vi "MathCad_Matrix_Get_string Elmnt.vi"(4 "row":i32, 6 "col":i32, 7 "error in":errorcluster, 8 "Mathcad.IMatrixValue Refnum":refnum<k7>, 9 "Worksheet Reference In":refnum<k7>) -> (0 "error out":errorcluster, 2 "Mathcad.IMatrixValue Refnum":refnum<k7>, 3 "Worksheet Reference Out":refnum<k7>, 5 "string":string)   [LabVIEW 2015]
doc: "Gets the value from the reference retrieved from the getrefnum VI."
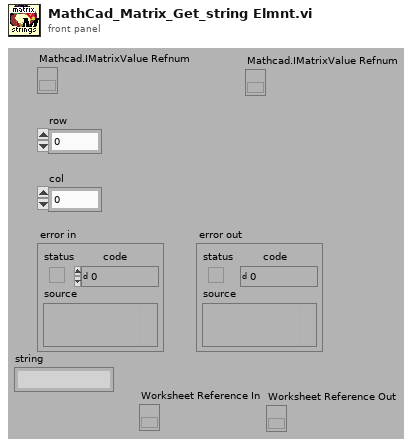
[diagram p1: front panel]
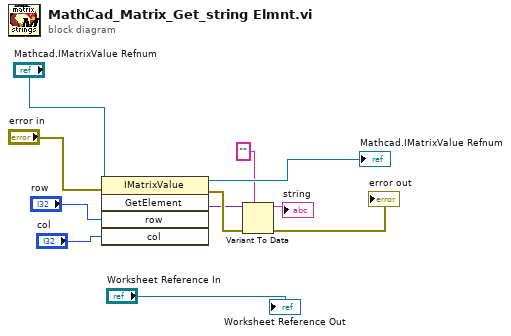
[diagram p0: block diagram]
diagram:
  n1 = invoke class="IMatrixValue" method="GetElement"(reference="Mathcad.IMatrixValue Refnum", error in="error in", "row"="row", "col"="col") -> (reference out=→"Mathcad.IMatrixValue Refnum":refnum<k7>, error out=w9:errorcluster, "GetElement"=w8:variant)  [unwired: 1 in, 2 out]
  n2 = Variant To Data(error in=w9, type="" ("data"), Variant=w8) -> (data=→"string":string, error out=→"error out":errorcluster)
  "Worksheet Reference Out" <- "Worksheet Reference In"
